vi "PIM Handle Strip Chart.vi"(7 "Strip by sample? (F = seconds)":bool, 8 "Strip Chart Display Data":T1, 11 "Measured PIM (dBm/dBc)":dbl[](array[numeric])) -> (0 "HistoryView?":bool, 1 "Strip Total Span (seconds|samples)":dbl, 2 "Strip Window Span (seconds|samples)":dbl, 3 "PIM Traces":cluster{"x-values":dbl[], "y-values":dbl[]}[](array[cluster]), 4 "Reset Clear?":bool, 5 "Point Plotted?":bool, 6 "Increment History?":bool)   [LabVIEW 2011]
uses:
  Strip Chart Display Data.ctl
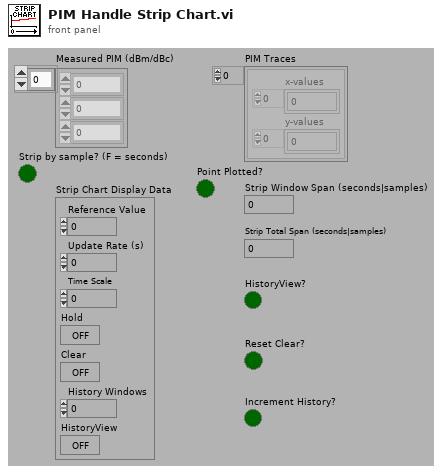
[diagram p1: front panel]
types:
  T1 = typedef "Strip Chart Display Data.ctl" = cluster{"Reference Value":dbl, "Update Rate (s)":dbl, "Time Scale":dbl, "Hold":bool, "Clear":bool, "History Windows":i32, "HistoryView":bool}
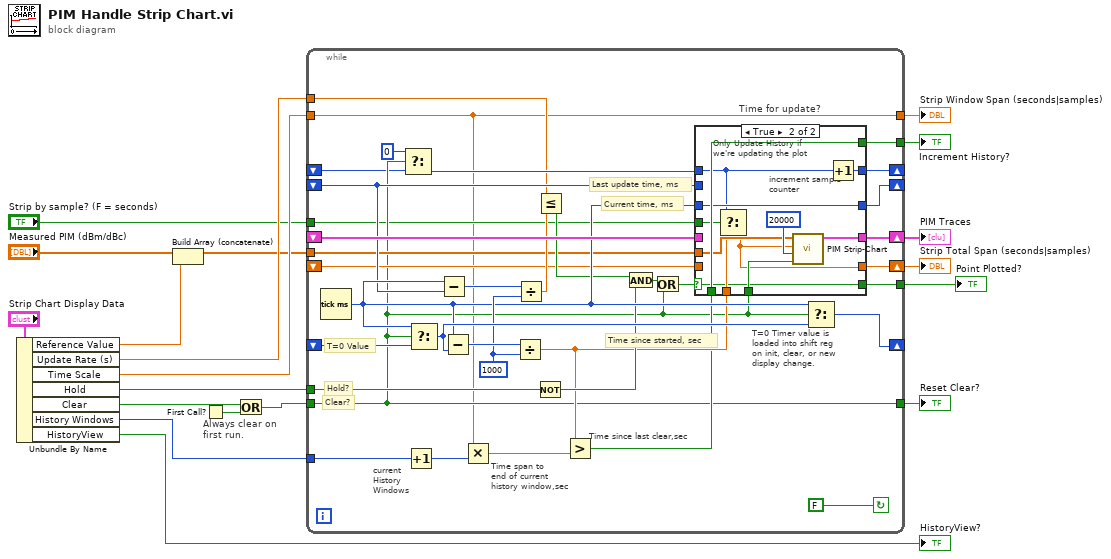
[diagram p0: block diagram]
diagram:
  # "Always clear on \nfirst run."
  n1 = Unbundle By Name("Strip Chart Display Data") -> ("Reference Value"=w4:dbl, "Update Rate (s)"=w11:dbl, "Time Scale"=w10:dbl, "Hold"=w9:bool, "Clear"=w8:bool, "History Windows"=w7:i32, "HistoryView"=→"HistoryView?":bool)
  n2 = Build Array (concatenate)("Measured PIM (dBm/dBc)", w4) -> (w3:dbl[])
  n3 = First Call?() -> (First Call?: T/F=w13:bool)
  n4 = Or(x=w8, y=w13) -> (x .or. y?=w12:bool)
  n5 = while {
    shift-left: _ -> [w38]
    shift-right: [w37] -> w16
    tunnel: w12 -> [w27]
    tunnel: w9 -> [w41]
    shift-left: _ -> [w44]
    shift-right: [w48] -> _
    tunnel: w11 -> [w22]
    shift-left: _ -> [w51]
    shift-right: [w53] -> w17
    shift-left: _ -> [w49]
    shift-right: [w54] -> _
    tunnel: w7 -> [w36]
    tunnel: [w27] -> w15
    tunnel: [w21] -> w18
    tunnel: [w30] -> w14
    tunnel: w10 -> [w21]
    tunnel: w3 -> [w29]
    shift-right: [w25] -> _
    shift-left: _ -> [w24]
    tunnel: "Strip by sample? (F = seconds)" -> [w23]
    tunnel: [w20] -> w1
    stop <- FALSE continue-if-true
    w46 = u32 1000 ("y")
    # "Time since last clear,sec"
    # "Time span to\nend of current\nhistory window,sec"
    # "current\nHistory\nWindows"
    # "Time since started, sec"
    # "T=0 Value"
    # "T=0 Timer value is\nloaded into shift reg\non init, clear, or new\ndisplay change."
    # "Clear?"
    # "Hold?"
    # "Current time, ms"
    # "Last update time, ms"
    n6 = Tick Count (ms)() -> (millisecond timer value=w45:u32)
    n7 = Select(t=0, s=w27, f=w24) -> (s? t:f=w26:i32)
    n8 = Increment(x=w36) -> (x+1=w35:i32)
    n9 = Select(t=w45, s=w27, f=w49) -> (s? t:f=w50:u32)
    n10 = Subtract(x=w45, y=w44) -> (x-y=w47:u32)
    n11 = Subtract(x=w45, y=w50) -> (x-y=w52:u32)
    n12 = Multiply(x=w21, y=w35) -> (x*y=w32:dbl)
    n13 = Divide(x=w52, y=w46) -> (x/y=w33:dbl)
    n14 = Divide(x=w47, y=w46) -> (x/y=w43:dbl)
    n15 = Not(x=w41) -> (.not. x?=w34:bool)
    n16 = Less Or Equal?(x=w22, y=w43) -> (x <= y?=w42:bool)
    n17 = Greater?(x=w33, y=w32) -> (0:w31:bool)
    n18 = And(x=w42, y=w34) -> (x .and. y?=w40:bool)
    n19 = Or(x=w40, y=w27) -> (x .or. y?=w39:bool)
    n20 = case "Time for update?" shown="True" w39 {
      selector: w39 -> [w56 w61]
      tunnel: w27 -> [_ w72]
      tunnel: [w60 w71] -> w53
      tunnel: w33 -> [_ w64]
      tunnel: w51 -> [w60 _]
      tunnel: w44 -> [w59 _]
      tunnel: [w59 w67] -> w48
      tunnel: w45 -> [_ w67]
      tunnel: w38 -> [w58 _]
      tunnel: [w58 w62] -> w37
      tunnel: w31 -> [_ w69]
      tunnel: [w56 w69] -> w30
      tunnel: w29 -> [_ w68]
      tunnel: w26 -> [w57 w65]
      tunnel: [w57 w66] -> w25
      tunnel: w23 -> [_ w63]
      tunnel: [w56 w61] -> w20
      frame False {
      }
      frame True {
        # "increment sample\ncounter"
        # "Only Update History if\nwe're updating the plot"
        n21 = Select(t=w65, s=w63, f=w64) -> (s? t:f=w62:dbl)
        n22 = call "PIM Strip-Chart.vi"("Clear Buffer (f)"=w72, "Buffer Length (2048)"=20000, "Update Time, sec"=w62, "Measured Values"=w68) -> ("Traces"=w71:cluster{"x-values":dbl[], "y-values":dbl[]}[])  [unwired: 3 out]
        n23 = Increment(x=w65) -> (x+1=w66:i32)
      }
    }
    n24 = Select(t=w45, s=w27, f=w50) -> (s? t:f=w54:u32)
  }
  "Strip Window Span (seconds|samples)" <- w18
  "PIM Traces" <- w17
  "Strip Total Span (seconds|samples)" <- w16
  "Reset Clear?" <- w15
  "Increment History?" <- w14
  "Point Plotted?" <- w1
